vi "GT_GetExtIoBit.vi"(3 "Index":i32, 4 "mdl":i32, 5 "rtn_In":cluster{"rtn":i16, "Func":string}) -> (1 "Status":bool, 2 "rtn_Out":cluster{"rtn":i16, "Func":string})   [LabVIEW 2014]
uses:
  data/data/ExtMdl.dll
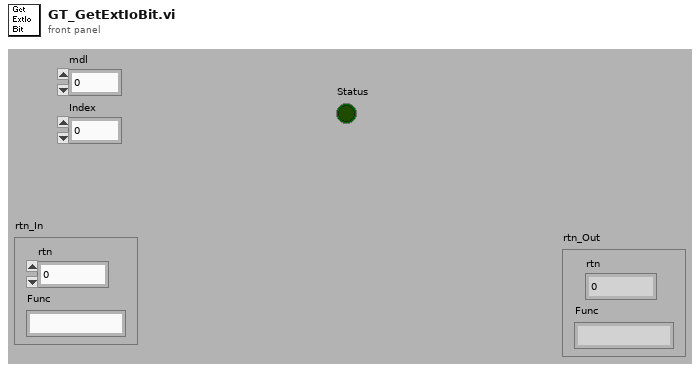
[diagram p1: front panel]
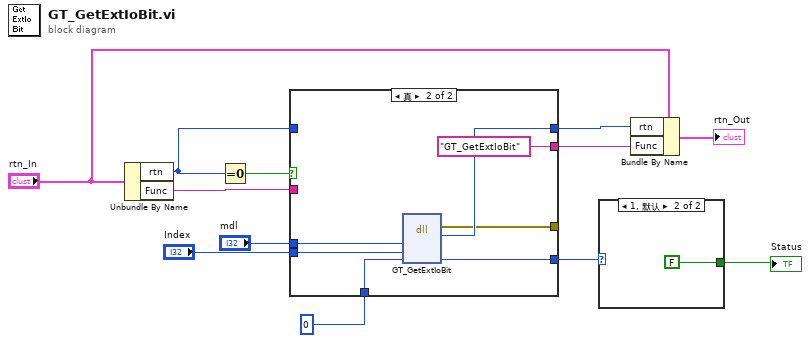
[diagram p0: block diagram]
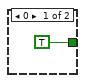
[diagram p2: hidden frame]
diagram:
  n1 = Unbundle By Name("rtn_In") -> ("rtn"=w10:i16, "Func"=w8:string)
  n2 = Equal To 0?(x=w10) -> (x = 0?=w12:bool)
  n3 = case shown="真" w12 {
    tunnel: w10 -> [w15 _]
    tunnel: [w15 w21] -> w9
    tunnel: w8 -> [w14 _]
    tunnel: [w14 "GT_GetExtIoBit" ("Func")] -> w7
    tunnel: [w13 w20] -> w2
    tunnel: "mdl" -> [_ w19]
    tunnel: "Index" -> [_ w18]
    tunnel: u32 0 ("pValue") -> [w13 w17]
    tunnel: [_ w16] -> _
    frame False {
    }
    frame True {
      n4 = dll-call lib="PTH2Sabs E\nSourceData&AC-800LWin7标准版源程序-20170923datadata\nExtMdl.dll" fn="GT_GetExtIoBit"("mdl"=w19, "Index"=w18, "pValue"=w17) -> (error out=w16:errorcluster, "rtn"=w21:i32, "pValue"=w20:u32)  [unwired: 5 in, 1 out]
    }
  }
  n5 = case shown="1, 默认" w2 {
    tunnel: [TRUE FALSE] -> w1
    frame 0 {
    }
    frame 1, Default {
    }
  }
  "Status" <- w1
  n6 = Bundle By Name(cluster="rtn_In", "rtn"=w9, "Func"=w7) -> (→"rtn_Out":cluster{"rtn":i16, "Func":string})
